vi "Shutter_Control.vi"(2 "error in":errorcluster, 3 "State":bool, 4 "Shutter":u16(ring) items=["Shutter Microscope", "Shutter Laser"]) -> (0 "error out":errorcluster)   [LabVIEW 2020]
uses:
  <vilib>/DAQmx/write.llb/DAQmx Write (Digital Bool 1Line 1Point).vi
  <vilib>/DAQmx/create/channels.llb/DAQmx Create Channel (DO-Digital Output).vi
  <vilib>/DAQmx/miscellaneous.llb/DAQmx Fill In Error Info.vi
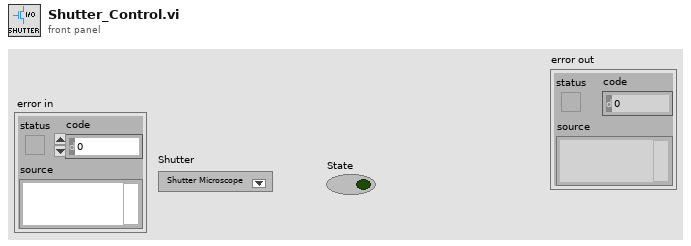
[diagram p1: front panel]
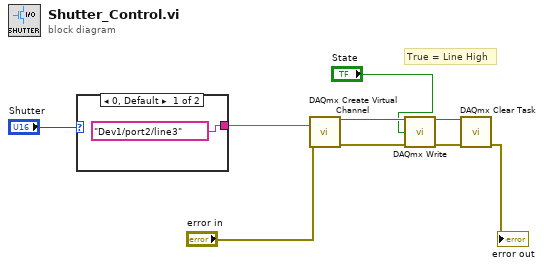
[diagram p0: block diagram]
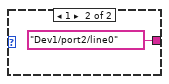
[diagram p2: hidden frame]
diagram:
  # "True = Line High"
  n1 = case shown="0, Default" "Shutter" {
    tunnel: [tag "Dev1/port2/line3" ("lines") tag "Dev1/port2/line0" ("lines")] -> w5
    frame 0, Default {
    }
    frame 1 {
    }
  }
  n2 = call-poly <vilib>:"DAQmx Create Virtual Channel.vi"("lines"=w5, "error in"="error in") -> ("task out"=w9:refnum<k21>, "error out"=w6:errorcluster)  [unwired: 12 in]
  n3 = call-poly <vilib>:"DAQmx Write.vi"("task/channels in"=w9, "data"="State", "error in"=w6) -> ("task out"=w8:refnum<k21>, "error out"=w7:errorcluster)  [unwired: 10 in, 1 out]
  n4 = call <vilib>:"DAQmx Clear Task.vi"("task in"=w8, "error in"=w7) -> ("error out"=→"error out":errorcluster)  [unwired: 13 in]
